vi "calc_r_jx.vi"(7 "index":i32, 11 "complex value":dbl[](array[numeric])) -> (3 "R+jX_Norm":cluster{"R":dbl, "jX":dbl})   [LabVIEW 2025]
panel:
  out "jX":dbl
  out "R":dbl
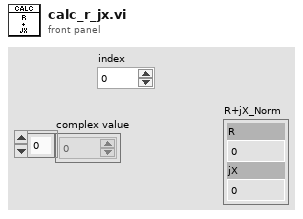
[diagram p1: front panel]
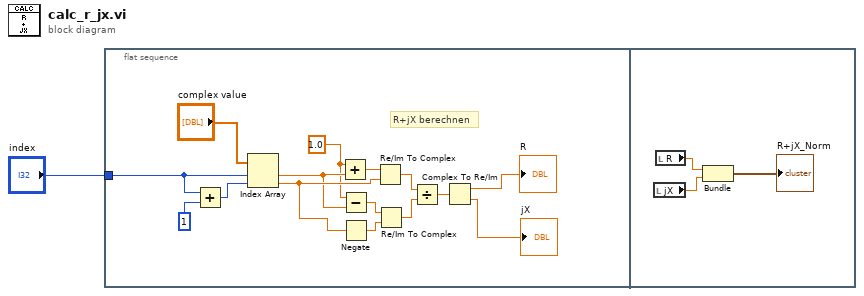
[diagram p0: block diagram]
diagram:
  n1 = flat-sequence {
    tunnel: "index" -> [w3]
    frame #0 {
      w5 = 1.0 ("x")
      # "R+jX berechnen"
      n2 = Add(x=w3, y=1) -> (x+y=w4:i32)
      n3 = Index Array(array="complex value", index #1=w3, index #2=w4) -> (element #1=w12:dbl, element #2=w14:dbl)
      n4 = Add(x=w5, y=w12) -> (x+y=w11:dbl)
      n5 = Subtract(x=w5, y=w12) -> (x-y=w10:dbl)
      n6 = Negate(x=w14) -> (-x=w9:dbl)
      n7 = Re/Im To Complex(1:w14, 2:w11) -> (0:w7:cdb)
      n8 = Re/Im To Complex(1:w9, 2:w10) -> (0:w8:cdb)
      n9 = Divide(x=w7, y=w8) -> (x/y=w6:cdb)
      n10 = Complex To Re/Im(x + iy=w6) -> (x=→"R":dbl, y=→"jX":dbl)
    }
    frame #1 {
      n11 = local read "jX"() -> (w18:dbl)
      n12 = local read "R"() -> (w17:dbl)
      n13 = Bundle("R"=w17, "jX"=w18) -> (→"R+jX_Norm":cluster{"R":dbl, "jX":dbl})  [unwired: 1 in]
    }
  }
